vi "W9EO82, FBO8PP_31.vi"() -> (3 "Array":i64[](array[numeric]))   [LabVIEW 2021]
uses:
  <vilib>/numeric/Random Number (Range) I64.vi
  <vilib>/numeric/sub_Random U32.vi
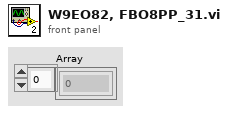
[diagram p1: front panel]
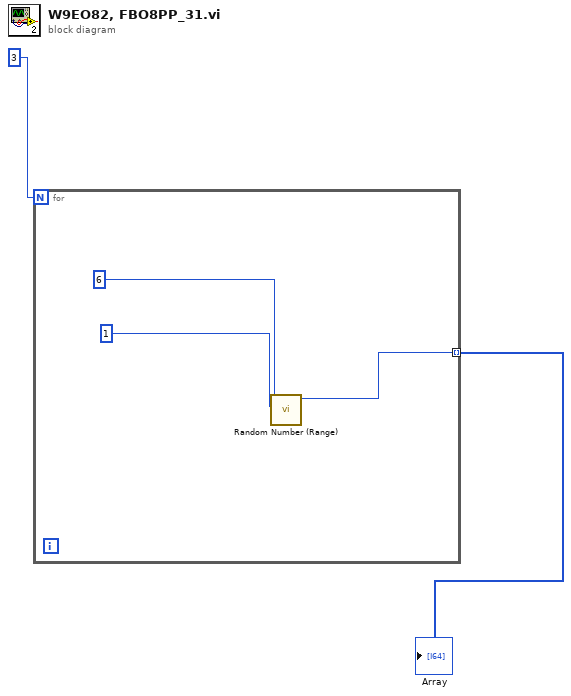
[diagram p0: block diagram]
diagram:
  n1 = for {
    N: 3 -> [_]
    tunnel: [w3] -> w1 mode=indexing
    n2 = call-poly <vilib>:"Random Number (Range).vi"("lower bound (-100)"=1, "upper bound (100)"=6) -> ("number"=w3:i64)  [unwired: 9 in]
  }
  "Array" <- w1
